vi "Untitled 1.vi"() -> ()   [LabVIEW 2018]
uses:
  <vilib>/AWS Toolkit/S3/Bucket/Bucket.lvclass
  <vilib>/AWS Toolkit/Core/HTTP Request/AWS Credentials.ctl
  <vilib>/AWS Toolkit/Core/HTTP Request/Region.ctl
  <vilib>/AWS Toolkit/S3/ACL.ctl
  <vilib>/AWS Toolkit/S3/GET Object Request Parameters.ctl
  <vilib>/AWS Toolkit/Core/Request Range.ctl
  <vilib>/AWS Toolkit/S3/GET Object Result Parameters.ctl
  <vilib>/AWS Toolkit/Core/HTTP Request/Name Value Pair.ctl
  <vilib>/AWS Toolkit/S3/NI_AWS_S3.lvlib
  <vilib>/AWS Toolkit/Core/HTTP Request/HTTP Request.lvclass
  <vilib>/AWS Toolkit/Core/NI_AWS_Core.lvlib
panel:
  out "error out 5":errorcluster
  out "User-Defined Metadata":T1[](array[typedef])
  out "Object Info":T2
  out "Data":string
  out "Bucket out 2":refnum<class "Bucket.lvclass">
  in  "Request Parameters":T3
  in  "Version ID":string
  in  "Object Path":string
  out "error out 4":errorcluster
  in  "Bucket Name":string
  out "Array":refnum<class "Bucket.lvclass">[](array[class])
  out "owner id":string
  out "owner display name":string
  out "error out 3":errorcluster
  in  "Access Control List":T5
  in  "Region":T6
  in  "AWS Credentials":T7
  in  "Name":string
  out "Bucket out":refnum<class "Bucket.lvclass">
  out "error out":errorcluster
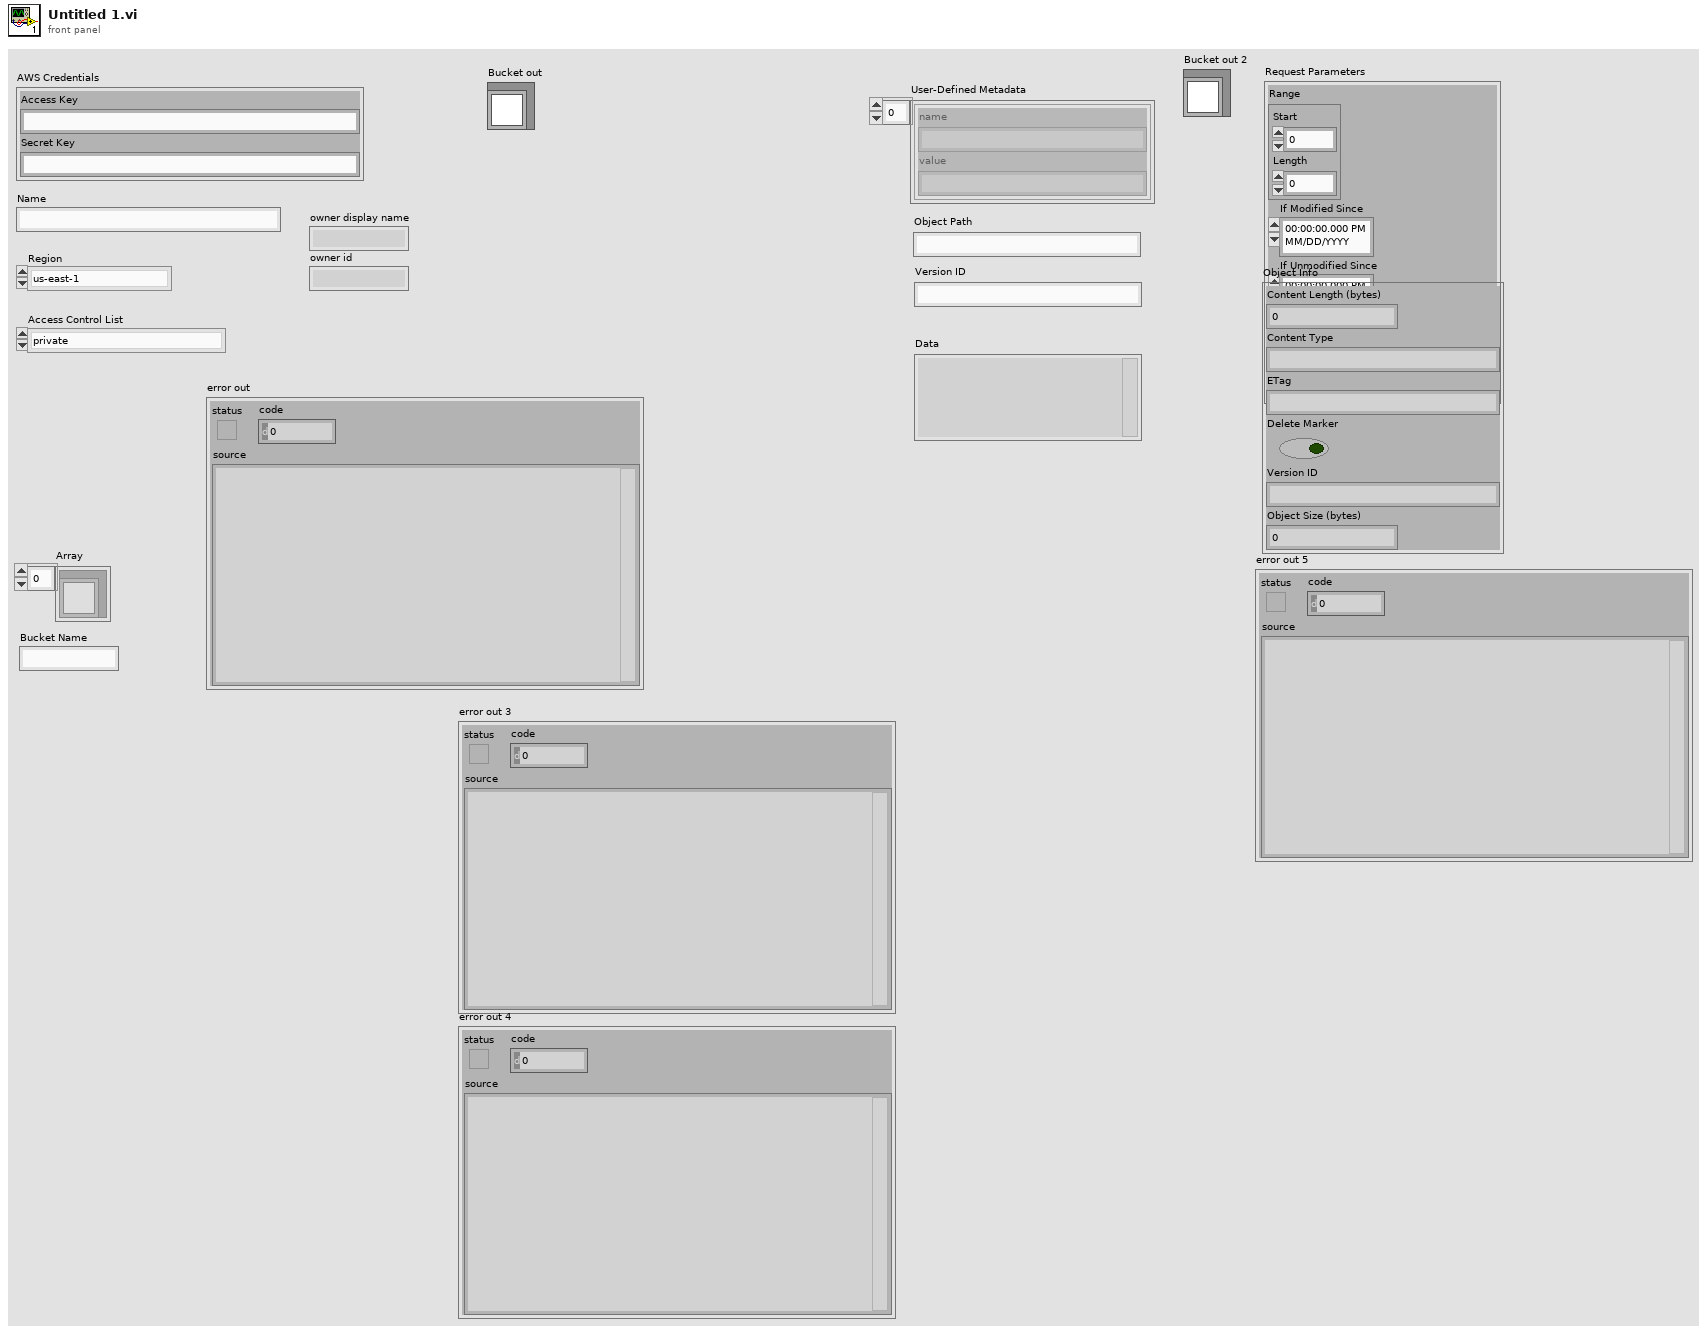
[diagram p1: front panel]
types:
  T1 = typedef "NI_AWS_Core.lvlib/HTTP Request.lvclass/Name Value Pair.ctl" = cluster{"name":string, "value":string}
  T2 = typedef "NI_AWS_S3.lvlib/GET Object Result Parameters.ctl" = cluster{"Content Length (bytes)":u64, "Content Type":string, "ETag":string, "Delete Marker":bool, "Version ID":string, "Object Size (bytes)":u64}
  T3 = typedef "NI_AWS_S3.lvlib/GET Object Request Parameters.ctl" = cluster{"Range":T4, "If Modified Since":timestamp, "If Unmodified Since":timestamp, "Matching ETag":string, "Nonmatching ETag":string}
  T4 = typedef "NI_AWS_Core.lvlib/Request Range.ctl" = cluster{"Start":i64, "Length":i64}
  T5 = typedef "NI_AWS_S3.lvlib/ACL.ctl" = enum16{"private", "public-read", "public-read-write", "aws-exec-read", "authenticated-read", "bucket-owner-read", "bucket-owner-full-control"}
  T6 = typedef "NI_AWS_Core.lvlib/HTTP Request.lvclass/Region.ctl" = enum16{"us-east-1", "us-east-2", "us-west-1", "us-west-2", "ap-northeast-1", "ap-northeast-2", "ap-southeast-1", "ap-southeast-2", "ca-central-1", "eu-central-1", "eu-west-1", "eu-west-2", "sa-east-1"}
  T7 = typedef "NI_AWS_Core.lvlib/HTTP Request.lvclass/AWS Credentials.ctl" = cluster{"Access Key":string, "Secret Key":string}
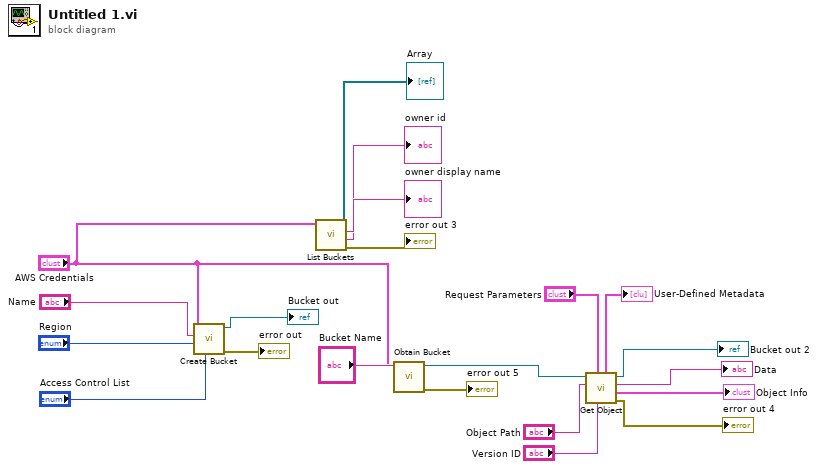
[diagram p0: block diagram]
diagram:
  n1 = call <vilib>:"Create Bucket.vi"("Access Control List"="Access Control List", "Region"="Region", "Name"="Name", "AWS Credentials"="AWS Credentials") -> ("error out"=→"error out":errorcluster, "Bucket out"=→"Bucket out":refnum<class "Bucket.lvclass">)  [unwired: 6 in]
  n2 = call <vilib>:"List Buckets.vi"("AWS Credentials"="AWS Credentials") -> ("error out"=→"error out 3":errorcluster, "Owner display name"=→"owner id":string, "Owner ID"=→"owner display name":string, "Buckets"=→"Array":refnum<class "Bucket.lvclass">[])  [unwired: 7 in]
  n3 = call <vilib>:"Obtain Bucket.vi"("Bucket name"="Bucket Name", "AWS Credentials"="AWS Credentials") -> ("error out"=→"error out 5":errorcluster, "Bucket"=w9:refnum<class "Bucket.lvclass">)  [unwired: 8 in]
  n4 = call <vilib>:"Get Object.vi"("Version ID"="Version ID", "Request Parameters"="Request Parameters", "Object Path"="Object Path", "Bucket in"=w9) -> ("error out"=→"error out 4":errorcluster, "Object Info"=→"Object Info":T2, "Data"=→"Data":string, "Bucket out"=→"Bucket out 2":refnum<class "Bucket.lvclass">, "User-Defined Metadata"=→"User-Defined Metadata":T1[])  [unwired: 3 in]
